vi "BRig_RT__Case_Exp__endTrial_checkFreeReward__v10.vi"(6 "input_dataBlock":u16[][](array[numeric]), 8 "input_dataExp":u16[](array[numeric]), 9 "input_dataTrial":u16[][](array[numeric]), 10 "input_dataCurrent":u16[](array[numeric])) -> (3 "output_state":T1, 5 "output_endBlock":bool)   [LabVIEW 2014]
uses:
  myRIO_BRig_RT__Case_Exp_stateList.ctl
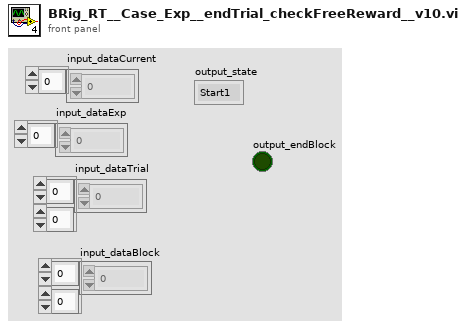
[diagram p1: front panel]
types:
  T1 = typedef "myRIO_BRig_RT__Case_Exp_stateList.ctl" = enum16{"Start1", "Start2", "Start3", "saveSettings1", "saveSettings2", "saveSettings3", "saveSettings4", "saveSettings_LC_ENL_l1", "saveSettings_LC_ENL_l2", "saveSettings_LC_Cue_l1", "saveSettings_LC_Cue_l2", "saveSettings6_LC_l1_Other", "SaveSettings6_LC_l2_Other", "setSettings_Audio", "setSettings_Laser", "initBlock_pre", "initBlock", "initBlock2", "initBlock_post", "initTrial_pre", "initTrial", "initTrial2", "initTrial3", "initTrial4", "initTrial_LC_ENL1", "initTrial_LC_Cue1", "initTrial_LC_Cue1_2", "initTrial_LC_Sel", "initTrial_post", "ENL1_pre", "ENL1", "ENL1_post", "ENL1Penalty_pre", "ENL1Penalty", "ENL2_pre", "ENL2", "ENL2Penalty_pre", "ENL2Penalty", "Cue1_pre", "Cue1", "Cue1_post", "Cue1Penalty_pre", "Cue1Penalty", "Cue2_pre", "Cue2", "Cue2Penalty_pre", "Cue2Penalty", "Selection_pre", "Selection", "Select_post", "SelectReward_pre", "SelectReward", "SelectRewardPost_pre", "SelectRewardPost", "SelectWrong_pre", "SelectWrong", "SelectWrong_post", "SelectTimeout_pre", "SelectTimeout", "SelectTimeout_post", "endTrial_pre", "endTrial1", "endTrial2", "endTrial3", "endTrial_post", "endBlock_pre", "endBlock", "endBlock_post", "endExp", "commConnect", "commUpload_pre", "commUpload_dataBlock", "commUpload_dataCurrent", "commUpload_dataExp", "commUpload_dataLC", "commUpload_dataTrial", "commUpload_post", "saveData_pre", "saveData_dataBlock", "saveData_dataCurrent", "saveData_dataExp", "saveData_dataLC", "saveData_dataTrial", "saveData_post", "empty_endBlock1", "empty_endBlock2", "empty_endTrial1", "empty_endTrial2", "empty_endTrial3", "empty_endTrial4", "empty_endTrial5", "dummyState", "dummyState_endBlock", "FreeReward_pre", "FreeReward", "FreeRewardPost_pre", "FreeRewardPost"}
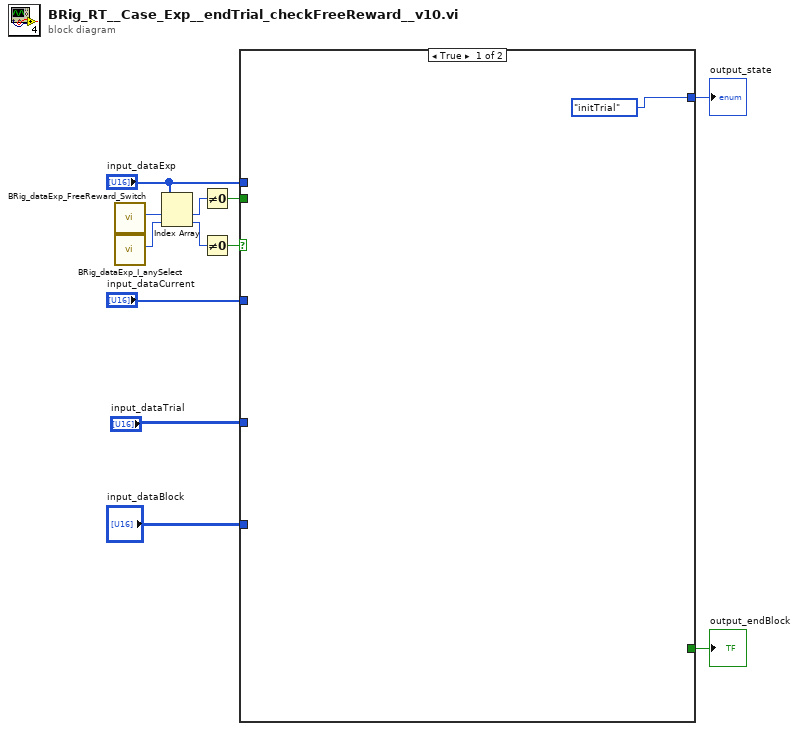
[diagram p0: block diagram]
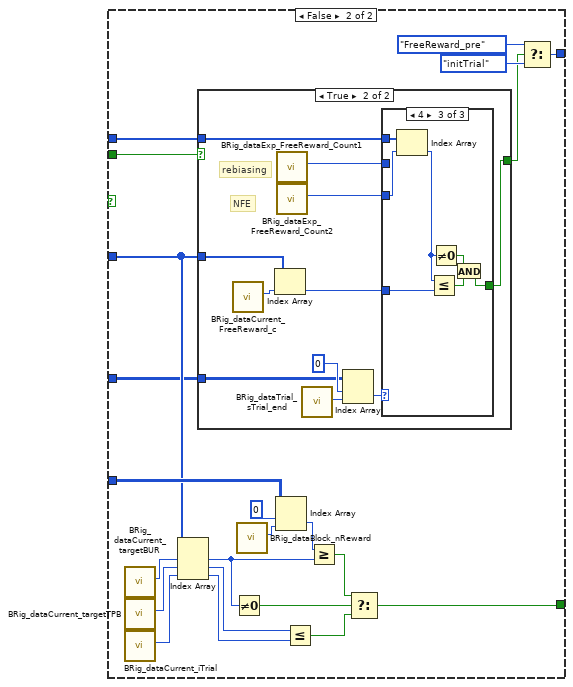
[diagram p2: hidden frame]
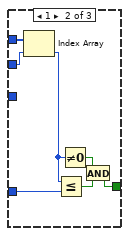
[diagram p5: hidden frame]
diagram:
  n1 = call "BRig_dataExp_FreeReward_Switch.vi"() -> ("output_FreeReward_Switch"=w12:i32)  [unwired: 11 in]
  n2 = call "BRig_dataExp_I_anySelect.vi"() -> ("output_I_anySelect"=w3:i32)  [unwired: 11 in]
  n3 = Index Array(array="input_dataExp", index #1=w12, index #2=w3) -> (element #1=w11:u16, element #2=w4:u16)
  n4 = Not Equal To 0?(x=w11) -> (x != 0?=w10:bool)
  n5 = Not Equal To 0?(x=w4) -> (x != 0?=w1:bool)
  n6 = case shown="True" w1 {
    tunnel: w10 -> [_ w33]
    tunnel: "input_dataExp" -> [_ w32]
    tunnel: [myRIO_BRig_RT__Case_Exp_stateList."initTrial" ("Enum") w30] -> w8
    tunnel: [_ w28] -> w7
    tunnel: "input_dataBlock" -> [_ w23]
    tunnel: "input_dataCurrent" -> [_ w15]
    tunnel: "input_dataTrial" -> [_ w14]
    frame True {
    }
    frame False {
      n7 = call "BRig_dataCurrent_targetBUR.vi"() -> ("output_targetBUR"=w17:i32)  [unwired: 11 in]
      n8 = call "BRig_dataCurrent_targetTPB.vi"() -> ("output_targetTPB"=w16:i32)  [unwired: 11 in]
      n9 = call "BRig_dataCurrent_iTrial.vi"() -> ("output_iTrial"=w18:i32)  [unwired: 11 in]
      n10 = Index Array(array=w15, index #1=w17, index #2=w16, index #3=w18) -> (element #1=w26:u16, element #2=w19:u16, element #3=w20:u16)
      n11 = case shown="True" w33 {
        selector: w33 -> [w36 _]
        tunnel: w32 -> [_ w44]
        tunnel: [w36 w40] -> w31
        tunnel: w15 -> [_ w38]
        tunnel: w14 -> [_ w37]
        frame False {
        }
        frame True {
          # "NFE"
          # "rebiasing"
          n12 = call "BRig_dataCurrent_FreeReward_c.vi"() -> ("output_FreeReward_c"=w47:i32)  [unwired: 11 in]
          n13 = Index Array(array=w38, index=w47) -> (element=w41:u16)
          n14 = call "BRig_dataExp_FreeReward_Count1.vi"() -> ("output_FreeReward_Count"=w43:i32)  [unwired: 11 in]
          n15 = call "BRig_dataExp_FreeReward_Count2.vi"() -> ("output_FreeReward_Count"=w42:i32)  [unwired: 11 in]
          n16 = call "BRig_dataTrial_sTrial_end.vi"() -> ("output_sTrial_end"=w46:i32)  [unwired: 11 in]
          n17 = Index Array(array=w37, index (row)=0, index (col)=w46) -> (element=w45:u16)
          n18 = case shown="4" w45 {
            tunnel: w44 -> [_ w54 w61]
            tunnel: w43 -> [_ w53 _]
            tunnel: w42 -> [_ _ w59]
            tunnel: w41 -> [_ w52 w60]
            tunnel: [_ w48 w55] -> w40
            frame 0, Default {
            }
            frame 1 {
              n19 = Index Array(array=w54, index=w53) -> (element=w51:u16)
              n20 = Less Or Equal?(x=w51, y=w52) -> (x <= y?=w50:bool)
              n21 = Not Equal To 0?(x=w51) -> (x != 0?=w49:bool)
              n22 = And(x=w49, y=w50) -> (x .and. y?=w48:bool)
            }
            frame 4 {
              n23 = Index Array(array=w61, index=w59) -> (element=w57:u16)
              n24 = Less Or Equal?(x=w57, y=w60) -> (x <= y?=w56:bool)
              n25 = Not Equal To 0?(x=w57) -> (x != 0?=w58:bool)
              n26 = And(x=w58, y=w56) -> (x .and. y?=w55:bool)
            }
          }
        }
      }
      n27 = Not Equal To 0?(x=w26) -> (x != 0?=w21:bool)
      n28 = call "BRig_dataBlock_nReward.vi"() -> ("output_nReward"=w24:i32)  [unwired: 11 in]
      n29 = Index Array(array=w23, index (row)=0, index (col)=w24) -> (element=w25:u16)
      n30 = Less Or Equal?(x=w19, y=w20) -> (x <= y?=w22:bool)
      n31 = Greater Or Equal?(x=w25, y=w26) -> (x >= y?=w27:bool)
      n32 = Select(t=w27, s=w21, f=w22) -> (s? t:f=w28:bool)
      n33 = Select(t=myRIO_BRig_RT__Case_Exp_stateList."FreeReward_pre" ("Enum"), s=w31, f=myRIO_BRig_RT__Case_Exp_stateList."initTrial" ("Enum")) -> (s? t:f=w30:T1)
    }
  }
  "output_state" <- w8
  "output_endBlock" <- w7
